vi "AVI-calculate split file frame index.vi"(8 "error in (no error)":errorcluster, 10 "Frame number (unity-based) in":i32=1 min=1, 11 "AVI modes refs":T2) -> (0 "error out":errorcluster, 1 "Index of frame in split file":u32, 2 "index of  split file":i32, 3 "AVI2 split file ref":T1)   [LabVIEW 2017]
uses:
  Typedefs/AVI modes refs cluster.ctl
  <vilib>/vision/Avi1.llb/AviRefnum.ctl
  <vilib>/vision/Avi.llb/IMAQ AVI2 Refnum.ctl
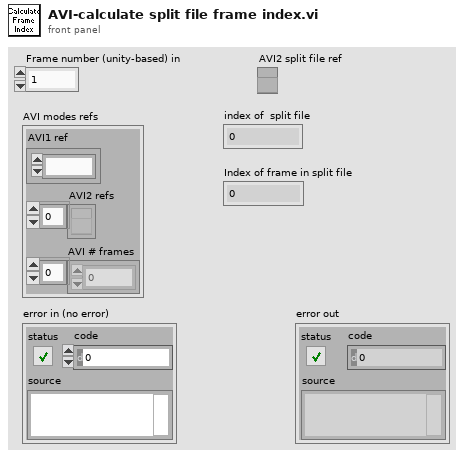
[diagram p1: front panel]
types:
  T1 = typedef "IMAQ AVI2 Refnum.ctl" = refnum<k20>
  T2 = typedef "AVI modes refs cluster.ctl" = cluster{"AVI1 ref":T3, "AVI2 refs":T1[], "AVI # frames":u32[]}
  T3 = typedef "AviRefnum.ctl" = refnum<k1>
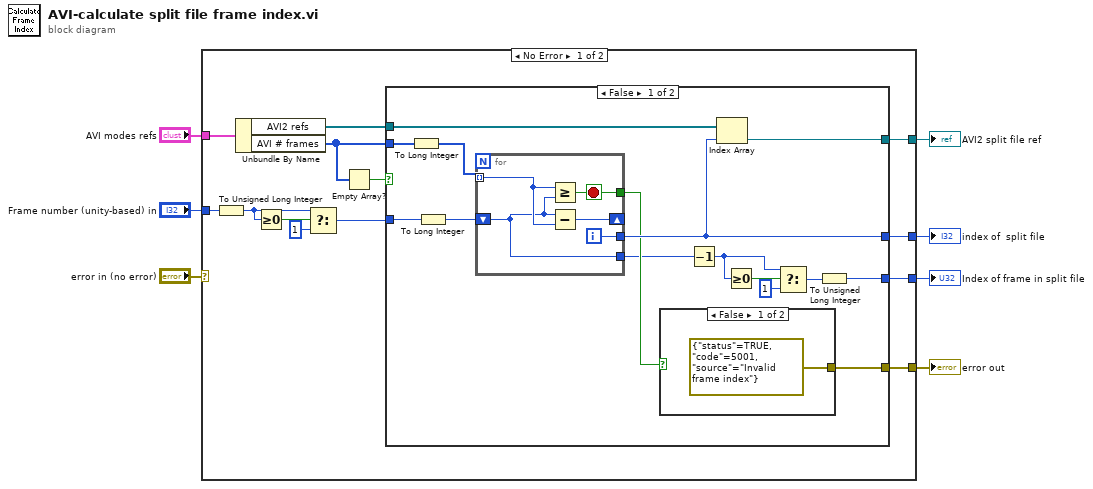
[diagram p0: block diagram]
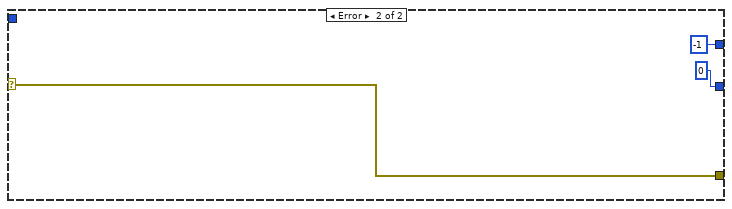
[diagram p4: hidden frame]
diagram:
  n1 = case shown="No Error" "error in (no error)" {
    selector: "error in (no error)" -> [_ w44]
    tunnel: "AVI modes refs" -> [w19 _]
    tunnel: [w18 _] -> w6
    tunnel: "Frame number (unity-based) in" -> [w15 _]
    tunnel: [w17 -1] -> w4
    tunnel: [w16 w44] -> w3
    tunnel: [w10 u32 0] -> w1
    frame No Error {
      n2 = To Unsigned Long Integer(number=w15) -> (unsigned 32bit integer=w12:u32)
      n3 = Unbundle By Name(w19) -> ("AVI2 refs"=w20:T1[], "AVI # frames"=w8:u32[])
      n4 = Greater Or Equal To 0?(x=w12) -> (x >= 0?=w14:bool)
      n5 = Select(t=w12, s=w14, f=u32 1) -> (s? t:f=w11:u32)
      n6 = Empty Array?(array=w8) -> (empty?=w9:bool)
      n7 = case shown="False" w9 {
        tunnel: w20 -> [w35 _]
        tunnel: [w34 _] -> w18
        tunnel: w8 -> [w33 _]
        tunnel: [w32 _] -> w17
        tunnel: [w30 _] -> w16
        tunnel: w11 -> [w24 _]
        tunnel: [w21 _] -> w10
        frame False {
          n8 = To Long Integer(number=w33) -> (32bit integer=w23:i32[])
          n9 = To Long Integer(number=w24) -> (32bit integer=w22:i32)
          n10 = for {
            tunnel: w23 -> [w39] mode=indexing
            tunnel: [w41] -> w32
            tunnel: [w40] -> w31
            shift-right: [w38] -> _
            shift-left: w22 -> [w37]
            tunnel: [w37] -> w29
            i -> [w41]
            stop <- w40 stop-if-true
            n11 = Greater Or Equal?(x=w39, y=w37) -> (x >= y?=w40:bool)
            n12 = Subtract(x=w37, y=w39) -> (x-y=w38:i32)
          }
          n13 = case shown="False" w31 {
            tunnel: [errorcluster {"status"=TRUE, "code"=5001, "source"="Invalid frame index"} ("error out") _] -> w30
            frame False {
            }
            frame True {
            }
          }
          n14 = Decrement(x=w29) -> (x-1=w26:i32)
          n15 = Index Array(array=w35, index=w32) -> (element=w34:T1)
          n16 = Greater Or Equal To 0?(x=w26) -> (x >= 0?=w28:bool)
          n17 = Select(t=w26, s=w28, f=1) -> (s? t:f=w25:i32)
          n18 = To Unsigned Long Integer(number=w25) -> (unsigned 32bit integer=w21:u32)
        }
        frame True {
          # "Prevents erroring out when used as a subVI in some of the\nfunctional data exporter's code."
        }
      }
    }
    frame Error {
    }
  }
  "Index of frame in split file" <- w1
  "index of  split file" <- w4
  "error out" <- w3
  "AVI2 split file ref" <- w6
